vi "practica112.vi"() -> ()   [LabVIEW 2017]
uses:
  <vilib>/Native 3D Graph/xcontrol/3DPC_SurfacePlot.xctl
panel:
  in  "S3":i32
  in  "eje z":dbl
  out "3D Graph":refnum<class "Base Datatype.lvclass">[](xcontrol)
  out "S2 x":dbl
  out "S2 y":dbl
  out "S1 x":dbl
  out "S1 y":dbl
  in  "S2":i32
  in  "S1":i32
  in  "stop":bool
  in  "S2":dbl(knob) scale=-175.0..175.0
  in  "S1":dbl(knob) scale=0.0..360.0
  out "XY Graph":cluster{"Y":dbl[], "Y":dbl[]}[](graph)
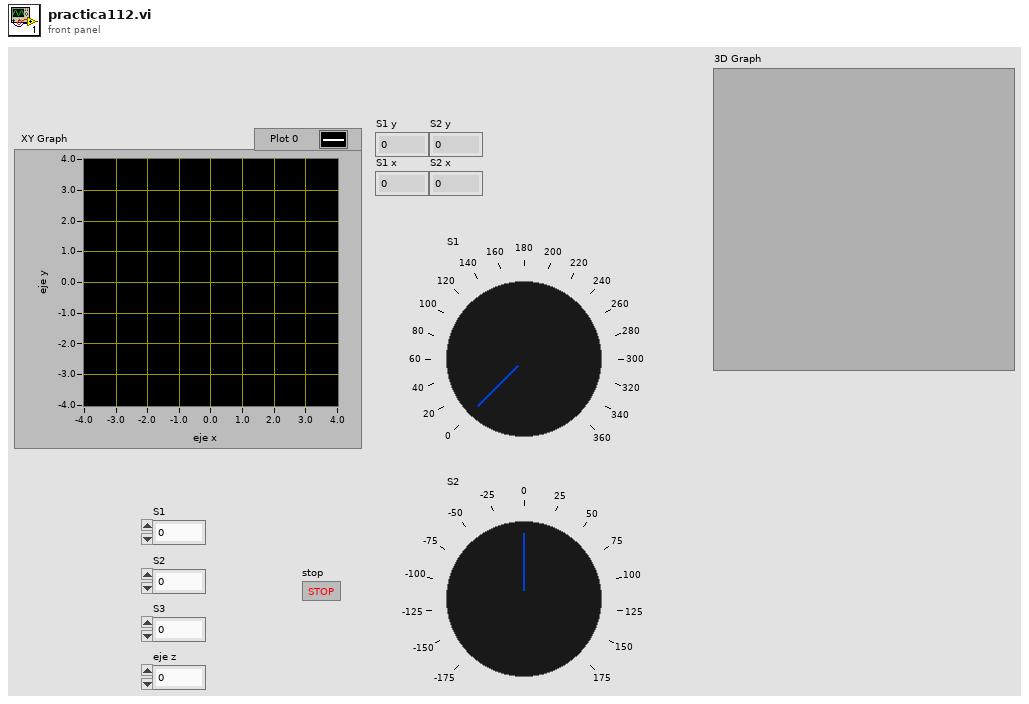
[diagram p1: front panel]
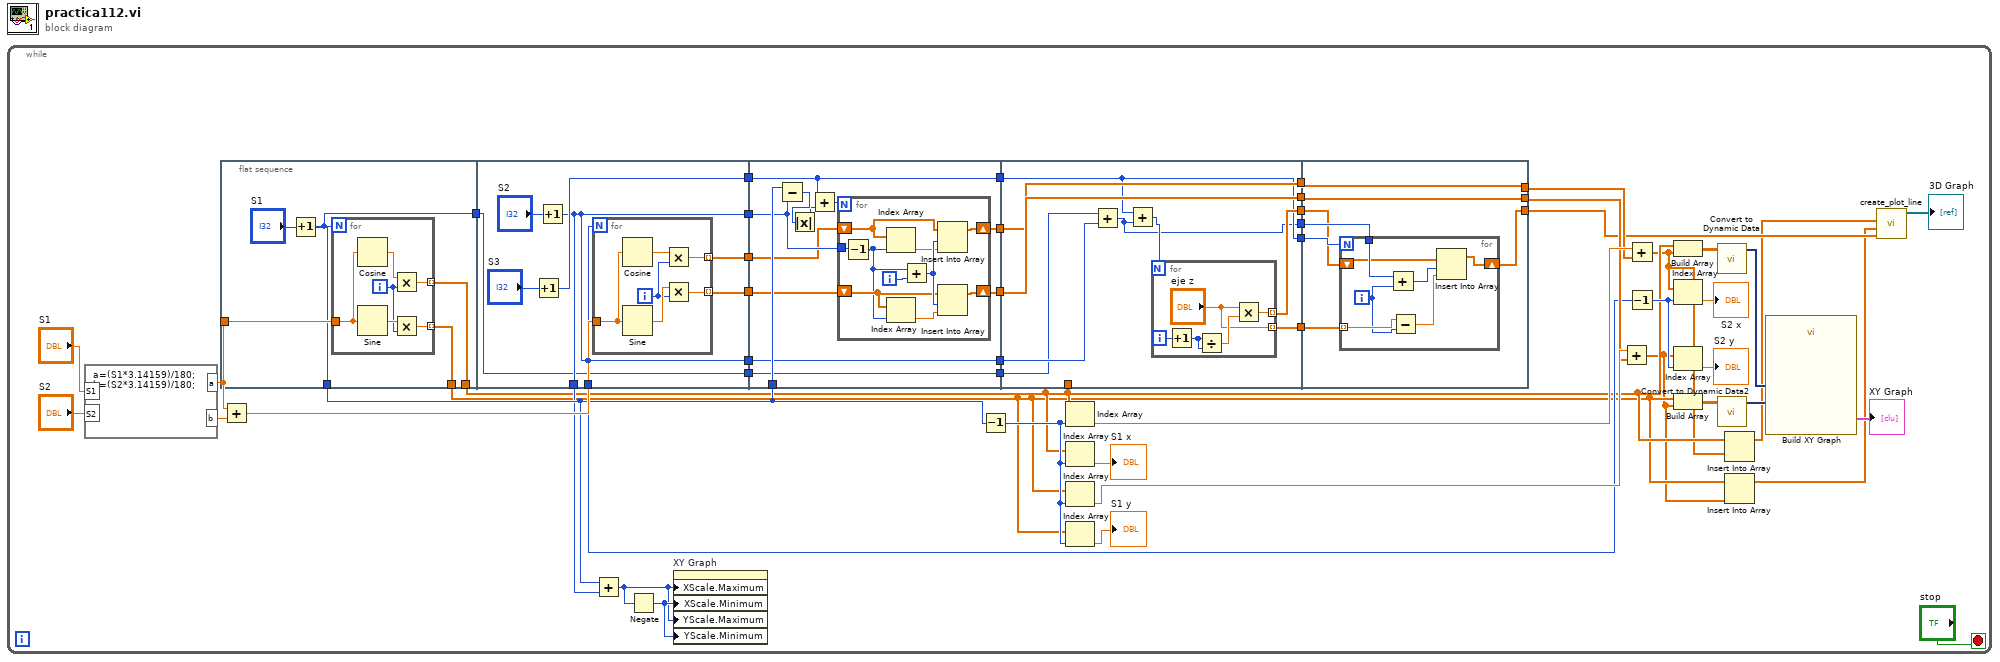
[diagram p0: block diagram]
diagram:
  n1 = while {
    stop <- "stop" stop-if-true
    n2 = formula code="a=(S1*3.14159)/180;\nb=(S2*3.14159)/180;"("S1"="S1", "S2"="S2") -> ("b"=w46:dbl, "a"=w45:dbl)
    n3 = flat-sequence {
      tunnel: w45 -> [w57]
      tunnel: [w53] -> w32
      tunnel: [w55] -> w17
      tunnel: [w54] -> w19
      tunnel: [w53] -> w5
      tunnel: w44 -> [w70]
      tunnel: [w69] -> w42
      tunnel: [w68] -> w41
      tunnel: [w65] -> w40
      tunnel: [w65] -> w33
      tunnel: [w65] -> w31
      tunnel: [w66] -> w10
      tunnel: [w65] -> w7
      tunnel: w5 -> [w64]
      tunnel: [w64] -> w4
      tunnel: w42 -> [w84]
      tunnel: w41 -> [w85]
      tunnel: w32 -> [w89]
      tunnel: w40 -> [w88]
      tunnel: [w86] -> w26
      tunnel: [w87] -> w25
      tunnel: w10 -> [w82]
      tunnel: [w82] -> w9
      tunnel: w7 -> [w81]
      tunnel: [w81] -> w6
      tunnel: w4 -> [w80]
      tunnel: [w80] -> w3
      tunnel: w26 -> [w107]
      tunnel: w25 -> [w108]
      tunnel: w19 -> [_]
      tunnel: [w107] -> w13
      tunnel: [w108] -> w12
      tunnel: [w106] -> w11
      tunnel: w9 -> [w102]
      tunnel: [w102] -> w8
      tunnel: w6 -> [w105]
      tunnel: w3 -> [w104]
      tunnel: [w103] -> w2
      tunnel: [w100] -> w1
      tunnel: [w115] -> w23
      tunnel: [w119] -> w37
      tunnel: [w120] -> w24
      tunnel: w13 -> [w120]
      tunnel: w12 -> [w119]
      tunnel: w11 -> [w116]
      tunnel: w8 -> [w118]
      tunnel: w2 -> [w114]
      tunnel: w1 -> [w117]
      frame #0 {
        n4 = Increment(x="S1") -> (x+1=w53:i32)
        n5 = for {
          N: w53 -> [_]
          tunnel: w57 -> [w59]
          tunnel: [w61] -> w55 mode=indexing
          tunnel: [w60] -> w54 mode=indexing
          i -> [w58]
          n6 = Cosine(x=w59) -> (cos(x)=w63:dbl)
          n7 = Sine(x=w59) -> (sin(x)=w62:dbl)
          n8 = Multiply(x=w63, y=w58) -> (x*y=w60:dbl)
          n9 = Multiply(x=w62, y=w58) -> (x*y=w61:dbl)
        }
      }
      frame #1 {
        n10 = Increment(x="S3") -> (x+1=w66:i32)
        n11 = Increment(x="S2") -> (x+1=w65:i32)
        n12 = for {
          N: w65 -> [_]
          tunnel: w70 -> [w73]
          tunnel: [w75] -> w68 mode=indexing
          tunnel: [w74] -> w69 mode=indexing
          i -> [w72]
          n13 = Cosine(x=w73) -> (cos(x)=w77:dbl)
          n14 = Sine(x=w73) -> (sin(x)=w76:dbl)
          n15 = Multiply(x=w77, y=w72) -> (x*y=w74:dbl)
          n16 = Multiply(x=w76, y=w72) -> (x*y=w75:dbl)
        }
      }
      frame #2 {
        n17 = Subtract(x=w89, y=w88) -> (x-y=w79:i32)
        n18 = Absolute Value(x=w79) -> (abs(x)=w78:i32)
        n19 = Add(x=w82, y=w78) -> (x+y=w83:i32)
        n20 = for {
          N: w83 -> [_]
          tunnel: w88 -> [w91]
          shift-right: [w95] -> w87
          shift-left: w85 -> [w97]
          shift-right: [w92] -> w86
          shift-left: w84 -> [w94]
          i -> [w99]
          n21 = Decrement(x=w91) -> (x-1=w90:i32)
          n22 = Index Array(array=w94, index=w90) -> (element=w93:dbl)
          n23 = Index Array(array=w97, index=w90) -> (element=w96:dbl)
          n24 = Add(x=w90, y=w99) -> (x+y=w98:i32)
          n25 = Insert Into Array(array=w94, index=w98, new element=w93) -> (w92:dbl[])
          n26 = Insert Into Array(array=w97, index=w98, new element=w96) -> (w95:dbl[])
        }
      }
      frame #3 {
        n27 = Add(x=w104, y=w105) -> (x+y=w100:i32)
        n28 = Add(x=w102, y=w100) -> (x+y=w101:i32)
        n29 = for {
          N: w101 -> [_]
          tunnel: [w112] -> w106 mode=indexing
          tunnel: ["eje z"] -> w103 mode=indexing
          i -> [w111]
          n30 = Increment(x=w111) -> (x+1=w110:i32)
          n31 = Divide(x=w110, y=w110) -> (x/y=w113:dbl)
          n32 = Multiply(x="eje z", y=w113) -> (x*y=w112:dbl)
        }
      }
      frame #4 {
        n33 = for {
          N: w118 -> [_]
          tunnel: w117 -> [w127]
          shift-right: [w122] -> w115
          shift-left: w116 -> [w125]
          tunnel: w114 -> [w124] mode=indexing
          i -> [w121]
          n34 = Add(x=w127, y=w121) -> (x+y=w126:i32)
          n35 = Subtract(x=w124, y=w121) -> (x-y=w123:dbl)
          n36 = Insert Into Array(array=w125, index=w126, new element=w123) -> (w122:dbl[])
        }
      }
    }
    n37 = Add(x=w45, y=w46) -> (x+y=w44:dbl)
    n38 = Add(x=w32, y=w31) -> (x+y=w29:i32)
    n39 = Negate(x=w29) -> (-x=w30:i32)
    n40 = property on="XY Graph" class="XYGraph (strict)"("XScale.Maximum"=w29, "XScale.Minimum"=w30, "YScale.Maximum"=w29, "YScale.Minimum"=w30) -> ()  [unwired: 2 in, 2 out]
    n41 = Decrement(x=w32) -> (x-1=w27:i32)
    n42 = Index Array(array=w19, index=w27) -> (element=w47:dbl)
    n43 = Index Array(array=w19, index=w27) -> (element=→"S1 x":dbl)
    n44 = Index Array(array=w17, index=w27) -> (element=w43:dbl)
    n45 = Index Array(array=w17, index=w27) -> (element=→"S1 y":dbl)
    n46 = Add(x=w43, y=w37) -> (x+y=w16:dbl[])
    n47 = Add(x=w47, y=w24) -> (x+y=w18:dbl[])
    n48 = Decrement(x=w33) -> (x-1=w34:i32)
    n49 = Build Array(w19, w18) -> (w22:dbl[][])
    n50 = Index Array(array=w18, index=w34) -> (element=→"S2 x":dbl)
    n51 = Index Array(array=w16, index=w34) -> (element=→"S2 y":dbl)
    n52 = Build Array(w17, w16) -> (w49:dbl[][])
    n53 = call "Convert to Dynamic Data"("2D Array"=w22) -> ("Dynamic Data Type"=w21:dynamicdata)  [unwired: 3 in]
    n54 = call "Convert to Dynamic Data2"("2D Array"=w49) -> ("Dynamic Data Type"=w20:dynamicdata)  [unwired: 3 in]
    n55 = Insert Into Array(array=w19, new element=w18) -> (w15:dbl[])  [unwired: 1 in]
    n56 = Insert Into Array(array=w17, new element=w16) -> (w14:dbl[])  [unwired: 1 in]
    n57 = call "Build XY Graph"("Y Input"=w20, "X Input"=w21) -> ("XY Graph"=→"XY Graph":cluster{"X":dbl[], "Y":dbl[]}[])  [unwired: 8 in, 1 out]
    n58 = call <vilib>:"create_plot_line.vi"("z vector"=w23, "y vector"=w14, "x vector"=w15) -> ("plots out"=→"3D Graph":refnum<class "Base Datatype.lvclass">[])  [unwired: 2 in, 6 out]
  }
